vi "Configure Selected Program.vi"(5 "Timeout (1 s)":dbl=1.0, 6 "Program Operation (0: Add Program Code)":i32(ring) items=["Add Program Code", "Define Program Code", "Delete All Programs", "Delete Selected Program", "Execute Program", "Change Execute Status", "Wait Until Status Changed"], 7 "Execution Status (0: Run)":i32(ring) items=["Run", "Pause", "Step", "Stop", "Continue"], 8 "error in (no error)":errorcluster, 9 "Program Name (program1)":string="program1", 10 "Program Code (#212:INP:STAT ON)":string="#212:INP:STAT ON", 11 "VISA resource name":refnum<visa-resource-name>) -> (0 "error out":errorcluster, 3 "VISA resource name out":refnum<visa-resource-name>)   [LabVIEW 2012, in "Keysight B2980 Series.lvlib"]
doc: "Configures the selected program to operate."
uses:
  Keysight B2980 Series.lvlib
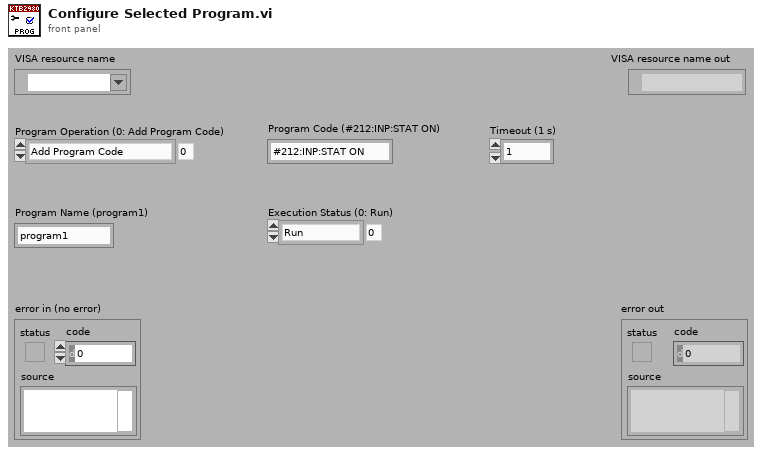
[diagram p1: front panel]
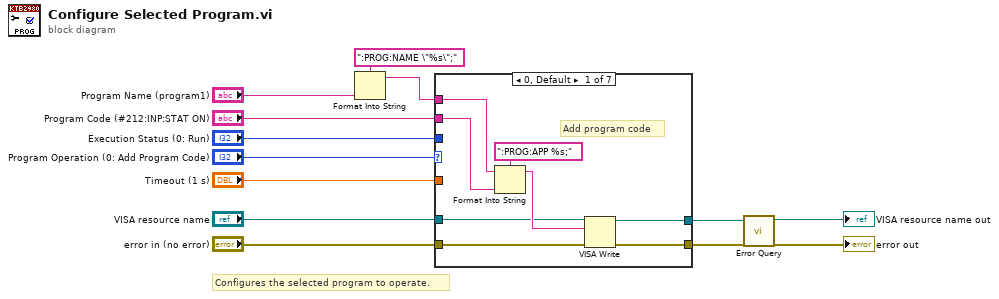
[diagram p0: block diagram]
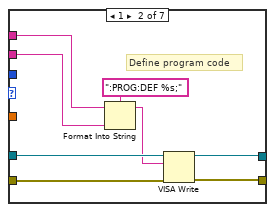
[diagram p2: hidden frame]
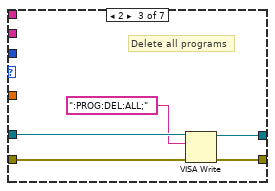
[diagram p3: hidden frame]
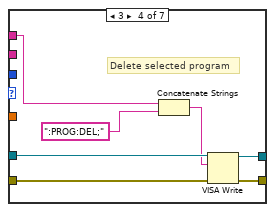
[diagram p4: hidden frame]
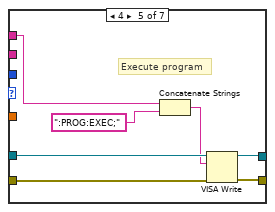
[diagram p5: hidden frame]
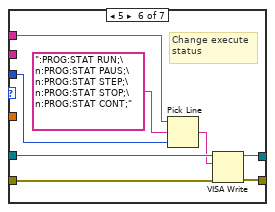
[diagram p6: hidden frame]
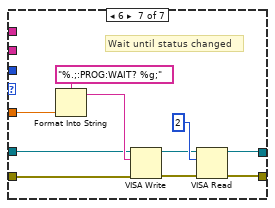
[diagram p7: hidden frame]
diagram:
  # "Configures the selected program to operate."
  n1 = Format Into String(format string=":PROG:NAME \"%s\";", "Program Name (program1)") -> (resulting string=w7:string)  [unwired: 2 in, 1 out]
  n2 = case shown="0, Default" "Program Operation (0: Add Program Code)" {
    tunnel: "Program Code (#212:INP:STAT ON)" -> [w20 w28 _ _ _ _ _]
    tunnel: w7 -> [w19 w27 _ w41 w48 w55 _]
    tunnel: "Execution Status (0: Run)" -> [_ _ _ _ _ w54 _]
    tunnel: "VISA resource name" -> [w17 w26 w34 w39 w46 w53 w61]
    tunnel: "error in (no error)" -> [w16 w24 w33 w38 w45 w52 w60]
    tunnel: [w15 w25 w31 w37 w43 w50 w59] -> w3
    tunnel: [w14 w23 w30 w36 w42 w49 w58] -> w2
    tunnel: "Timeout (1 s)" -> [_ _ _ _ _ _ w57]
    frame 0, Default {
      # "Add program code"
      n3 = Format Into String(format string=":PROG:APP %s;", initial string=w19, w20) -> (resulting string=w18:string)  [unwired: 1 in, 1 out]
      n4 = VISA Write(VISA resource name=w17, write buffer=w18, error in (no error)=w16) -> (VISA resource name out=w15:refnum<visa-resource-name>, error out=w14:errorcluster)  [unwired: 1 out]
    }
    frame 1 {
      # "Define program code"
      n5 = Format Into String(format string=":PROG:DEF %s;", initial string=w27, w28) -> (resulting string=w22:string)  [unwired: 1 in, 1 out]
      n6 = VISA Write(VISA resource name=w26, write buffer=w22, error in (no error)=w24) -> (VISA resource name out=w25:refnum<visa-resource-name>, error out=w23:errorcluster)  [unwired: 1 out]
    }
    frame 2 {
      # "Delete all programs"
      n7 = VISA Write(VISA resource name=w34, write buffer=":PROG:DEL:ALL;", error in (no error)=w33) -> (VISA resource name out=w31:refnum<visa-resource-name>, error out=w30:errorcluster)  [unwired: 1 out]
    }
    frame 3 {
      # "Delete selected program"
      n8 = Concatenate Strings(w41, ":PROG:DEL;") -> (w35:string)
      n9 = VISA Write(VISA resource name=w39, write buffer=w35, error in (no error)=w38) -> (VISA resource name out=w37:refnum<visa-resource-name>, error out=w36:errorcluster)  [unwired: 1 out]
    }
    frame 4 {
      # "Execute program"
      n10 = Concatenate Strings(w48, ":PROG:EXEC;") -> (w44:string)
      n11 = VISA Write(VISA resource name=w46, write buffer=w44, error in (no error)=w45) -> (VISA resource name out=w43:refnum<visa-resource-name>, error out=w42:errorcluster)  [unwired: 1 out]
    }
    frame 5 {
      # "Change execute\nstatus"
      n12 = Pick Line(string ("")=w55, multi-line string=":PROG:STAT RUN;\n:PROG:STAT PAUS;\n:PROG:STAT STEP;\n:PROG:STAT STOP;\n:PROG:STAT CONT;", line index=w54) -> (output string=w51:string)
      n13 = VISA Write(VISA resource name=w53, write buffer=w51, error in (no error)=w52) -> (VISA resource name out=w50:refnum<visa-resource-name>, error out=w49:errorcluster)  [unwired: 1 out]
    }
    frame 6 {
      # "Wait until status changed"
      n14 = Format Into String(format string="%.;:PROG:WAIT? %g;", w57) -> (resulting string=w63:string)  [unwired: 2 in, 1 out]
      n15 = VISA Write(VISA resource name=w61, write buffer=w63, error in (no error)=w60) -> (VISA resource name out=w64:refnum<visa-resource-name>, error out=w65:errorcluster)  [unwired: 1 out]
      n16 = VISA Read(VISA resource name=w64, byte count=u32 2, error in (no error)=w65) -> (VISA resource name out=w59:refnum<visa-resource-name>, error out=w58:errorcluster)  [unwired: 2 out]
    }
  }
  n17 = call "Error Query.vi"("error in (no error)"=w2, "VISA resource name"=w3) -> ("error out"=→"error out":errorcluster, "VISA resource name out"=→"VISA resource name out":refnum<visa-resource-name>)  [unwired: 8 out]
